vi "interface_configure.vi"(8 "error in (no error)":errorcluster, 11 "configuration in":T1) -> (0 "error out":errorcluster, 3 "configuration out":T1)   [LabVIEW 2015, in "lv-build-interface.lvlib"]
uses:
  lv-build-interface.lvlib
  lv-build/public/_controls/configuration.ctl
  <vilib>/Utility/error.llb/Error Cluster From Error Code.vi
  <vilib>/ErrorRing/Error Ring.xnode
  lv-build/lv-build.lvlib
panel:
  in  "cancel":bool
  in  "save":bool
  in  "distribution_folder":path caption="Distribution Folder"
  in  "dependencies_folder":path caption="Dependencies Folder"
  in  "bin_path":path caption="Bin Path"
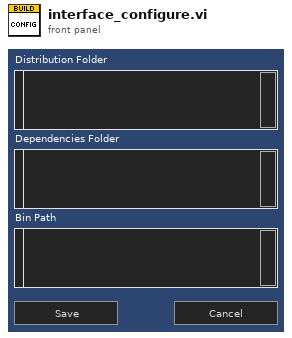
[diagram p1: front panel]
types:
  T1 = typedef "lv-build.lvlib/configuration.ctl" = cluster{"project_file":string, "distribution_folder":string, "dependencies_folder":string, "build_class_file":string, "version":string, "bin_path":string}
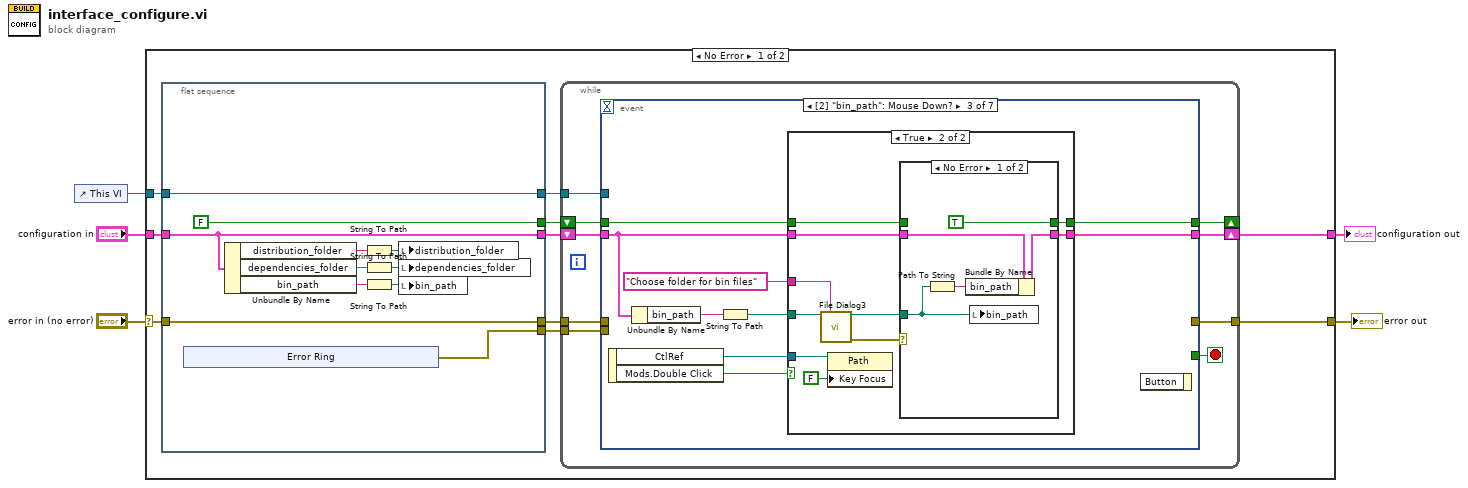
[diagram p0: block diagram]
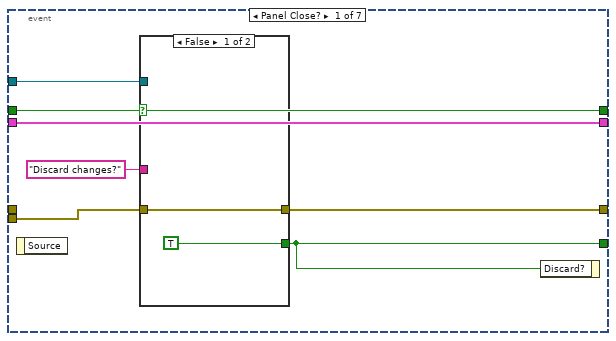
[diagram p2: hidden frame]
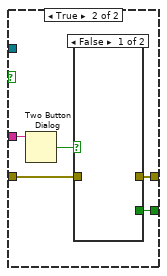
[diagram p3: hidden frame]
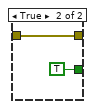
[diagram p4: hidden frame]
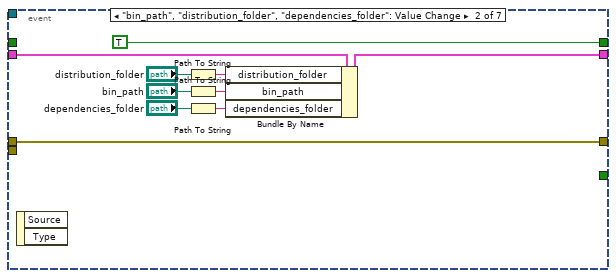
[diagram p5: hidden frame]
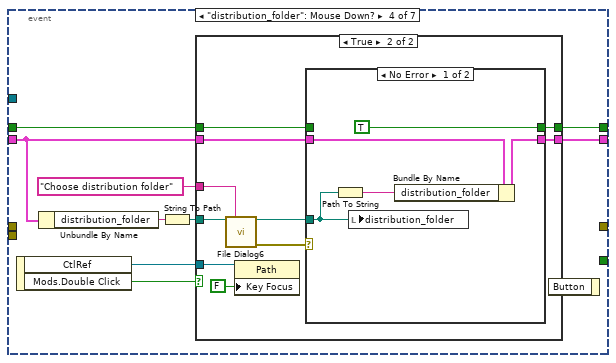
[diagram p8: hidden frame]
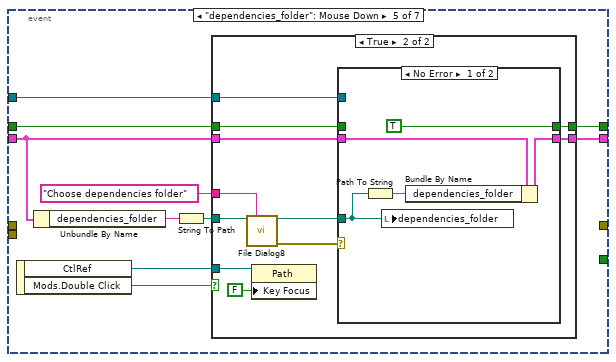
[diagram p11: hidden frame]
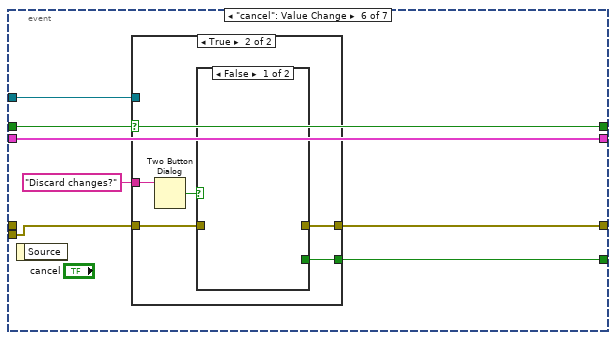
[diagram p14: hidden frame]
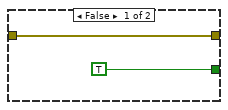
[diagram p15: hidden frame]
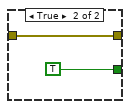
[diagram p16: hidden frame]
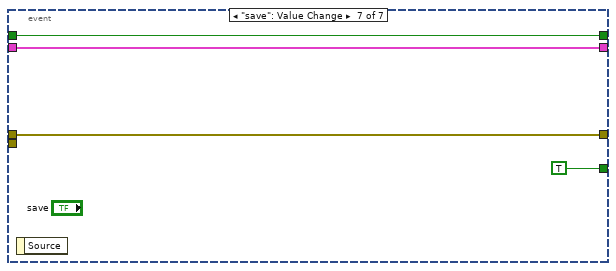
[diagram p17: hidden frame]
diagram:
  n1 = control-ref of="This VI"() -> (w3:refnum<vi>)
  n2 = case shown="No Error" "error in (no error)" {
    selector: "error in (no error)" -> [w15 w172]
    tunnel: [w9 w172] -> w4
    tunnel: w3 -> [w11 _]
    tunnel: [w8 _] -> w1
    tunnel: "configuration in" -> [w7 _]
    frame No Error {
      n3 = flat-sequence {
        tunnel: w15 -> [w20]
        tunnel: [w20] -> w14
        tunnel: [w21] -> w13
        tunnel: [w25] -> w12
        tunnel: w11 -> [w25]
        tunnel: [FALSE] -> w10
        tunnel: w7 -> [w21]
        tunnel: [w16] -> w6
        frame #0 {
          n4 = xnode "Error Ring"() -> ("error out"=w16:errorcluster)
          n5 = Unbundle By Name(w21) -> ("distribution_folder"=w19:string, "dependencies_folder"=w18:string, "bin_path"=w17:string)
          n6 = String To Path(string=w19) -> (path=w23:path)
          n7 = String To Path(string=w18) -> (path=w22:path)
          n8 = String To Path(string=w17) -> (path=w24:path)
          n9 = local write "distribution_folder"(w23) -> ()
          n10 = local write "dependencies_folder"(w22) -> ()
          n11 = local write "bin_path"(w24) -> ()
        }
      }
      n12 = while {
        tunnel: w14 -> [w32]
        shift-right: [w37] -> w8
        shift-left: w13 -> [w38]
        tunnel: w12 -> [w34]
        shift-right: [w35] -> _
        shift-left: w10 -> [w36]
        tunnel: [w33] -> w9
        tunnel: w6 -> [w31]
        stop <- w39 stop-if-true
        n13 = event shown="[2] \"bin_path\": Mouse Down?" {
          selector: _ -> [_ _ _ _ _ _ _]
          dyn-events: _ -> [_ _ _ _ _ _ _]
          timeout: _ -> [_ _ _ _ _ _ _]
          tunnel: [w44 _ _ _ _ w158 TRUE ("Discard?")] -> w39
          tunnel: w34 -> [w43 _ _ _ w127 w156 _]
          tunnel: w38 -> [w46 w65 w70 w98 w126 w157 w170]
          tunnel: [w46 w63 w72 w100 w129 w157 w170] -> w37
          tunnel: w36 -> [w42 _ w74 w102 w131 w154 w171]
          tunnel: [w42 TRUE w73 w101 w130 w154 w171] -> w35
          tunnel: [w41 w56 _ _ _ w152 w169] -> w33
          tunnel: w32 -> [_ w56 _ _ _ _ w169]
          tunnel: w31 -> [w40 _ _ _ _ w153 _]
          event Panel Close? {
            n14 = event-data() -> ()  [unwired: 1 in, 1 out]
            n15 = case shown="False" w42 {
              tunnel: [TRUE ("Discard?") w53] -> w44
              tunnel: w43 -> [_ _]
              tunnel: "Discard changes?" ("dialog_text") -> [_ w52]
              tunnel: [w47 w50] -> w41
              tunnel: w40 -> [w47 w49]
              frame False {
              }
              frame True {
                n16 = Two Button Dialog(message=w52) -> (T button?=w51:bool)  [unwired: 2 in]
                n17 = case shown="False" w51 {
                  tunnel: [_ TRUE ("Discard?")] -> w53
                  tunnel: [_ w54] -> w50
                  tunnel: w49 -> [_ w54]
                  frame False {
                  }
                  frame True {
                  }
                }
              }
            }
            n18 = event-data("Discard?"=w44) -> ()  [unwired: 1 in, 1 out]
          }
          event "bin_path", "distribution_folder", "dependencies_folder": Value Change {
            n19 = event-data() -> ()  [unwired: 1 in, 2 out]
            n20 = Path To String(path="distribution_folder") -> (string=w59:string)
            n21 = Path To String(path="bin_path") -> (string=w58:string)
            n22 = Path To String(path="dependencies_folder") -> (string=w57:string)
            n23 = Bundle By Name(cluster=w65, "distribution_folder"=w59, "bin_path"=w58, "dependencies_folder"=w57) -> (w63:T1)
          }
          event "bin_path": Mouse Down? {
            n24 = event-data() -> ("CtlRef"=w66:refnum<vi>, "Mods.Double Click"=w71:bool)  [unwired: 1 in]
            n25 = Unbundle By Name(w70) -> ("bin_path"=w69:string)
            n26 = String To Path(string=w69) -> (path=w67:path)
            n27 = case shown="True" w71 {
              tunnel: w74 -> [w76 w86]
              tunnel: w70 -> [w75 w85]
              tunnel: [w76 w84] -> w73
              tunnel: [w75 w83] -> w72
              tunnel: w67 -> [_ w81]
              tunnel: "Choose folder for bin files" ("description") -> [_ w82]
              tunnel: w66 -> [_ w77]
              frame False {
              }
              frame True {
                n28 = call "File Dialog3"("start path"=w81, "prompt"=w82) -> ("selected path"=w80:path, "error out"=w79:errorcluster)  [unwired: 10 in, 2 out]
                n29 = property on="Property Node" class="Path"(reference=w77, "Key Focus"=FALSE) -> ()  [unwired: 1 in, 2 out]
                n30 = case shown="No Error" w79 {
                  tunnel: w86 -> [_ w93]
                  tunnel: w85 -> [w90 w92]
                  tunnel: [TRUE w93] -> w84
                  tunnel: [w89 w92] -> w83
                  tunnel: w80 -> [w88 _]
                  frame No Error {
                    n31 = Path To String(path=w88) -> (string=w87:string)
                    n32 = Bundle By Name(cluster=w90, "bin_path"=w87) -> (w89:T1)
                    n33 = local write "bin_path"(w88) -> ()
                  }
                  frame Error {
                  }
                }
              }
            }
            n34 = event-data() -> ()  [unwired: 2 in, 1 out]
          }
          event "distribution_folder": Mouse Down? {
            n35 = event-data() -> ("CtlRef"=w94:refnum<vi>, "Mods.Double Click"=w99:bool)  [unwired: 1 in]
            n36 = Unbundle By Name(w98) -> ("distribution_folder"=w97:string)
            n37 = String To Path(string=w97) -> (path=w95:path)
            n38 = case shown="True" w99 {
              tunnel: w102 -> [w104 w114]
              tunnel: w98 -> [w103 w113]
              tunnel: [w104 w112] -> w101
              tunnel: [w103 w111] -> w100
              tunnel: w95 -> [_ w109]
              tunnel: "Choose distribution folder" ("description") -> [_ w108]
              tunnel: w94 -> [_ w105]
              frame False {
              }
              frame True {
                n39 = call "File Dialog6"("start path"=w109, "prompt"=w108) -> ("selected path"=w110:path, "error out"=w107:errorcluster)  [unwired: 10 in, 2 out]
                n40 = property on="Property Node" class="Path"(reference=w105, "Key Focus"=FALSE) -> ()  [unwired: 1 in, 2 out]
                n41 = case shown="No Error" w107 {
                  tunnel: w114 -> [_ w121]
                  tunnel: w113 -> [w118 w120]
                  tunnel: [TRUE w121] -> w112
                  tunnel: [w117 w120] -> w111
                  tunnel: w110 -> [w116 _]
                  frame No Error {
                    n42 = Path To String(path=w116) -> (string=w115:string)
                    n43 = local write "distribution_folder"(w116) -> ()
                    n44 = Bundle By Name(cluster=w118, "distribution_folder"=w115) -> (w117:T1)
                  }
                  frame Error {
                  }
                }
              }
            }
            n45 = event-data() -> ()  [unwired: 2 in, 1 out]
          }
          event "dependencies_folder": Mouse Down {
            n46 = event-data() -> ("CtlRef"=w122:refnum<vi>, "Mods.Double Click"=w128:bool)  [unwired: 1 in]
            n47 = Unbundle By Name(w126) -> ("dependencies_folder"=w125:string)
            n48 = String To Path(string=w125) -> (path=w123:path)
            n49 = case shown="True" w128 {
              tunnel: w131 -> [w133 w144]
              tunnel: w126 -> [w132 w143]
              tunnel: [w133 w142] -> w130
              tunnel: [w132 w141] -> w129
              tunnel: w127 -> [_ w140]
              tunnel: w123 -> [_ w139]
              tunnel: "Choose dependencies folder" ("description") -> [_ w136]
              tunnel: w122 -> [_ w134]
              frame False {
              }
              frame True {
                n50 = call "File Dialog8"("start path"=w139, "prompt"=w136) -> ("selected path"=w138:path, "error out"=w137:errorcluster)  [unwired: 10 in, 2 out]
                n51 = property on="Property Node" class="Path"(reference=w134, "Key Focus"=FALSE) -> ()  [unwired: 1 in, 2 out]
                n52 = case shown="No Error" w137 {
                  tunnel: w144 -> [_ w151]
                  tunnel: w143 -> [w148 w150]
                  tunnel: [TRUE w151] -> w142
                  tunnel: [w147 w150] -> w141
                  tunnel: w138 -> [w146 _]
                  tunnel: w140 -> [_ _]
                  frame No Error {
                    n53 = Path To String(path=w146) -> (string=w145:string)
                    n54 = local write "dependencies_folder"(w146) -> ()
                    n55 = Bundle By Name(cluster=w148, "dependencies_folder"=w145) -> (w147:T1)
                  }
                  frame Error {
                  }
                }
              }
            }
          }
          event "cancel": Value Change {
            n56 = event-data() -> ()  [unwired: 1 in, 1 out]
            n57 = case shown="True" w154 {
              tunnel: [TRUE ("Discard?") w165] -> w158
              tunnel: w156 -> [_ _]
              tunnel: "Discard changes?" ("dialog_text") -> [_ w163]
              tunnel: w153 -> [w159 w162]
              tunnel: [w159 w161] -> w152
              frame False {
              }
              frame True {
                n58 = Two Button Dialog(message=w163) -> (T button?=w164:bool)  [unwired: 2 in]
                n59 = case shown="False" w164 {
                  tunnel: [_ TRUE ("Discard?")] -> w165
                  tunnel: w162 -> [_ w166]
                  tunnel: [_ w166] -> w161
                  frame False {
                  }
                  frame True {
                  }
                }
              }
            }
          }
          event "save": Value Change {
            n60 = event-data() -> ()  [unwired: 1 in, 1 out]
          }
        }
      }
    }
    frame Error {
    }
  }
  "error out" <- w4
  "configuration out" <- w1
